vi "Set State Factory.vi"(10 "stateFactory":refnum<class "State Factory.lvclass">, 11 "Model in":refnum<class "Model.lvclass">) -> (3 "Model out":refnum<class "Model.lvclass">)   [LabVIEW 2015, in "Model.lvclass"]
uses:
  Model.lvclass
  States/State Factory/State Factory.lvclass
  Model.lvclass/Model.ctl
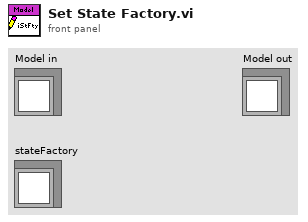
[diagram p1: front panel]
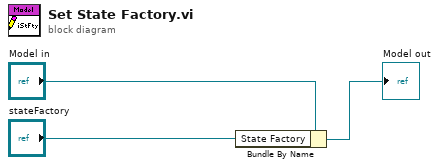
[diagram p0: block diagram]
diagram:
  n1 = Bundle By Name(cluster="Model in", "State Factory"="stateFactory") -> (→"Model out":refnum<class "Model.lvclass">)
